vi "Get RichText RTF.vi"(8 "error in (no error)":errorcluster caption="错误输入（无错误）", 11 "RichText 输入":refnum<class "RichText.lvclass"> caption="DNL_LabVIEW Object in") -> (0 "error out":errorcluster caption="错误输出", 2 "Rtf":string, 3 "RichText 输出":refnum<class "RichText.lvclass"> caption="DNL_LabVIEW Object out")   [LabVIEW 2012, in "RichText.lvclass"]
uses:
  RichText.lvclass
  RichText.lvclass/RichText.ctl
  System.Windows.Forms
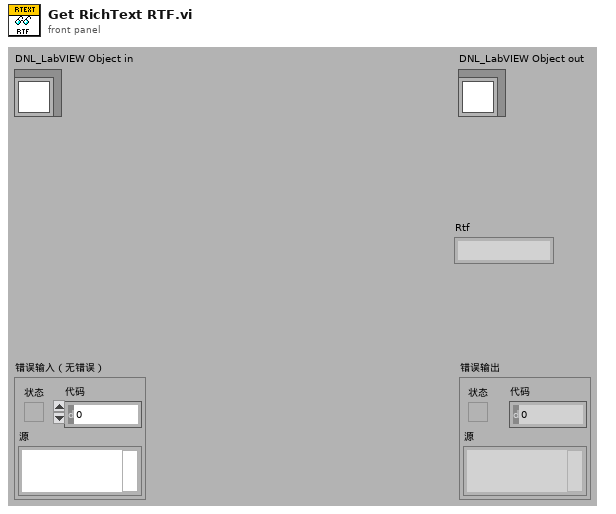
[diagram p1: front panel]
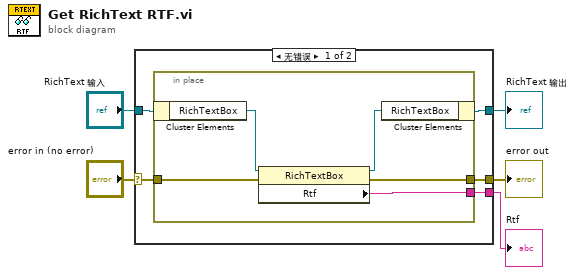
[diagram p0: block diagram]
diagram:
  n1 = case shown="无错误" "error in (no error)" {
    selector: "error in (no error)" -> [w9 w17]
    tunnel: [w6 w17] -> w4
    tunnel: [w7 w16] -> w2
    tunnel: "RichText 输入" -> [w10 w16]
    tunnel: [w8 _] -> w1
    frame No Error {
      n2 = in-place {
        in-place-border: w9 -> [w13]
        in-place-border: [w12] -> w8
        in-place-border: [w11] -> w6
        n3 = in-place-cluster #1(w10) -> ("RichTextBox"=w15:refnum<k24>)
        n4 = property class="RichTextBox"(reference=w15, error in=w13) -> (reference out=w14:refnum<k24>, error out=w11:errorcluster, "Rtf"=w12:string)
        n5 = in-place-cluster #1("RichTextBox"=w14) -> (w7:refnum<class "RichText.lvclass">)
      }
    }
    frame Error {
    }
  }
  "error out" <- w4
  "RichText 输出" <- w2
  "Rtf" <- w1
